vi "Delaunay.vi"(8 "error in (no error)":errorcluster, 11 "points":dbl[][](array[numeric])) -> (0 "error out":errorcluster, 3 "simplices":i32[][](array[numeric]))   [LabVIEW 2023, in "QHull.lvlib"]
uses:
  QHull.lvlib
  LV_QHull_64.dll
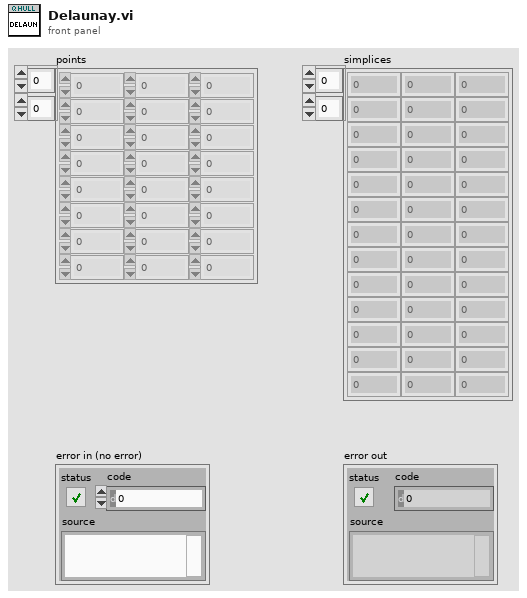
[diagram p1: front panel]
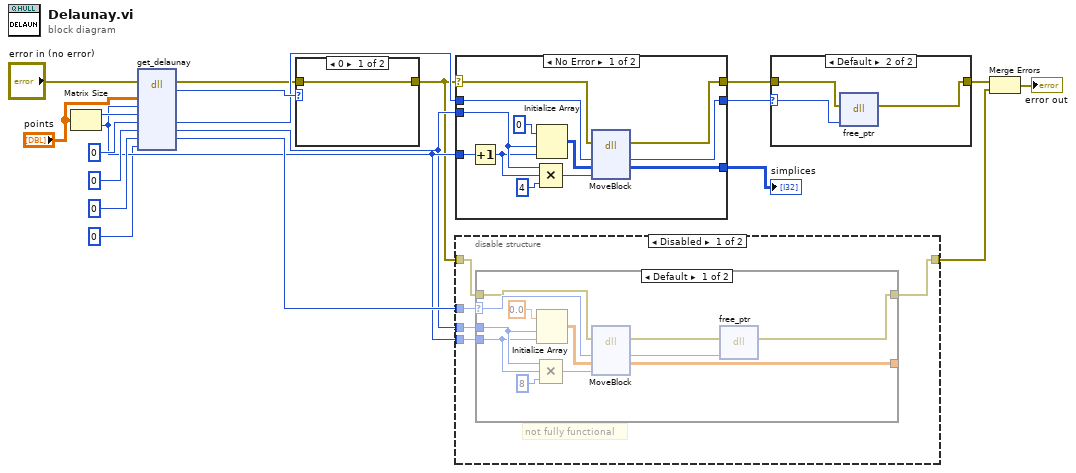
[diagram p0: block diagram]
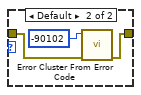
[diagram p5: hidden frame]
diagram:
  n1 = Matrix Size(0:"points") -> (1:w17:i32, 2:w8:i32)
  n2 = dll-call lib="E:/Labview/LV 2023/PPL/PPL Builder/Libs/SK Spatial/QHull/LV QHull/LV_QHull**.dll" fn="get_delaunay"(error in="error in (no error)", "points"="points", "dim"=w8, "numpoints"=w17, "simplices"=i64 0, "numsimplices"=0, "centers"=i64 0, "voronoi"=0) -> (error out=w5:errorcluster, "errorcode"=w14:i32, "simplices"=w9:i64, "numsimplices"=w7:i32, "centers"=w10:i64)  [unwired: 6 in, 1 out]
  n3 = case shown="0" w14 {
    tunnel: w5 -> [w21 w24]
    tunnel: [w21 w23] -> w4
    frame 0 {
    }
    frame Default {
      n4 = call <vilib>:"Error Cluster From Error Code.vi"("error in (no error)"=w24, "error code (0)"=-90102) -> ("error out"=w23:errorcluster)  [unwired: 7 in]
    }
  }
  n5 = case shown="No Error" w4 {
    selector: w4 -> [w28 w38]
    tunnel: w9 -> [w35 w37]
    tunnel: w8 -> [w34 _]
    tunnel: w7 -> [w32 _]
    tunnel: [w27 _] -> w15
    tunnel: [w26 w37] -> w13
    tunnel: [w25 w38] -> w12
    frame No Error {
      n6 = Increment(x=w34) -> (x+1=w31:i32)
      n7 = Initialize Array(0 ("element"), w32, w31) -> (w33:i32[][])
      n8 = Compound Arithmetic op=MULTIPLY(w32, w31, 4 ("value")) -> (w29:i32)
      n9 = dll-call lib="LabVIEW" fn="MoveBlock"(error in=w28, "ps"=w35, "pd"=w33, "size"=w29) -> (error out=w25:errorcluster, "ps"=w26:i64, "pd"=w27:i32[][])  [unwired: 4 in, 1 out]
    }
    frame Error {
    }
  }
  "simplices" <- w15
  n10 = disable-structure shown="Disabled" {
    disable-tunnel: w10 -> [w43 _]
    disable-tunnel: w8 -> [w42 _]
    disable-tunnel: w7 -> [w41 _]
    disable-tunnel: [w40 w57] -> w6
    disable-tunnel: w4 -> [w39 w57]
    frame Disabled {
      # "not fully functional"
      n11 = case shown="Default" w43 {
        selector: w43 -> [w54 _]
        tunnel: w41 -> [w52 _]
        tunnel: [w48 _] -> _
        tunnel: [w44 w56] -> w40
        tunnel: w42 -> [w47 _]
        tunnel: w39 -> [w49 w56]
        frame Default {
          n12 = Initialize Array(0.0 ("element"), w52, w47) -> (w53:dbl[][])
          n13 = Compound Arithmetic op=MULTIPLY(w52, w47, 8 ("value")) -> (w50:i32)
          n14 = dll-call lib="LabVIEW" fn="MoveBlock"(error in=w49, "ps"=w54, "pd"=w53, "size"=w50) -> (error out=w46:errorcluster, "ps"=w45:i64, "pd"=w48:dbl[][])  [unwired: 4 in, 1 out]
          n15 = dll-call lib="E:/Labview/LV 2023/PPL/PPL Builder/Libs/SK Spatial/QHull/LV QHull/LV_QHull**.dll" fn="free_ptr"(error in=w46, "ptr"=w45) -> (error out=w44:errorcluster)  [unwired: 4 in, 1 out]
        }
        frame 0 {
        }
      }
    }
    frame Enabled {
    }
  }
  n16 = case shown="Default" w13 {
    selector: w13 -> [_ w59]
    tunnel: w12 -> [w58 w61]
    tunnel: [w58 w60] -> w2
    frame 0 {
    }
    frame Default {
      n17 = dll-call lib="E:/Labview/LV 2023/PPL/PPL Builder/Libs/SK Spatial/QHull/LV QHull/LV_QHull**.dll" fn="free_ptr"(error in=w61, "ptr"=w59) -> (error out=w60:errorcluster)  [unwired: 4 in, 1 out]
    }
  }
  n18 = Merge Errors(w2, w6) -> (→"error out":errorcluster)
